vi "TLB Native Dynamic Events ver 0.08d beta.vi"() -> ()   [LabVIEW 2018]
uses:
  Labview Training Phase 2/Enum Controls/States for Action Engine.ctl
  Type def/TLB event states.ctl
  Type def/TLB MHL States.ctl
  <vilib>/Studica/Studica Toolkit/Background/I2C Channel.ctl
  <vilib>/myRIO/Common/Instrument Driver Framework/myRIO v1.0/AI/typedefs/AI Channels Enum.ctl
  <vilib>/myRIO/Common/Instrument Driver Framework/myRIO v1.0/AI/typedefs/AI Channels List.ctl
  Type def/Type def.ctl
  <vilib>/Studica/Studica Blackhawk/Blackhawk.lvlib
  <vilib>/Studica/Studica Toolkit/Background/Mxp Selection.ctl
  <vilib>/Studica/Studica Toolkit/Background/DIO Channel.ctl
  <vilib>/NI_Real-Time Target Support.lvlib
  <vilib>/ptbypt/NI_PtbyPt.lvlib
  <vilib>/addons/control/pid/NI_PID_pid.lvlib
  Underlying VI's/Webcam FGV Low level ver/State control.ctl
  <vilib>/userdefined/High Color/IMAQdx.ctl
  <vilib>/Studica/Studica Toolkit/NavX/NavX.lvlib
  <vilib>/addons/control/pid/pid.llb/PID (DBL).vi
  <vilib>/Studica/Studica Toolkit/NavX/TypeDefs/Flags/Z900_navX_Flags_CalibrationStatusTypeDef.ctl
  <vilib>/Studica/Studica Toolkit/NavX/TypeDefs/Flags/Z900_navX_Flags_OpStatusTypeDef.ctl
panel:
  out "Sensor loop error":errorcluster
  out "Status":T3 {"OP Status" items=["INITIALIZING", "SELFTEST_IN_PROGRESS", "ERROR", "IMU_AUTOCAL_IN_PROGRESS", "NORMAL"]; "Calibration Status" items=["IMU_CAL_STATE_MASK"=3, "IMU_CAL_STATE_INPROGRESS"=0, "IMU_CAL_STATE_ACCUMULATE"=1, "IMU_CAL_STATE_COMPLETE"=2]}
  out "NavX error":errorcluster
  out "Arduino error":errorcluster
  in  "Data to Write":u8[](array[numeric])
  out "Displacement":T4
  out "Yaw":dbl
  out "Speed and distance cluster":T5
  out "Output":dbl
  in  "SENSOR":bool
  out "Decision":i8
  out "Manual Zero Yaw":bool
  in  "error in (no error)":errorcluster
  in  "RED LED State":enum16{"OFF", "ON", "BLINK"}(ring)
  in  "GREEN LED State":enum16{"OFF", "ON", "BLINK"}(ring)
  in  "Red LED":bool
  in  "Green LED":bool
  out "Input state":i8
  out "Waveform Chart 2":dbl(graph)
  out "Waveform Chart":dbl(graph)
  in  "STOP":bool
  out "DIO 0":bool
  out "DIO 1":bool
  out "Limit Switch Array":bool[](array[boolean])
  out "error out":errorcluster
  out "L/R average":fxp<+,64,64>
  out "Right Ultrasonic":fxp<+,64,16>
  out "Left Ultrasonic":fxp<+,64,16>
  out "Right IR Sensor":dbl
  out "Left IR Sensor":dbl
  out "Object detection count":T6
  out "Camera error":errorcluster
  in  "Servo Angle":u8(slide) scale=0.0..180.0
  in  "On/Off":bool
  out "Blackhawk error":errorcluster
  out "element":T7
  out "Action Queue Items":i32
  out "State Logic Queue Items":i32
  out "Action Queues items":string[](array[string])=["Hardware reset", "Software reset", ""]
  out "State logic":T8=enum."Task 2"
  out "Action State":string
  # "TLB FRAMEWORK STATUS"
  # "Camera Status Loop"
  # "Test Programme written by Calvin Loke    Dated: 28 Aug 2019\nTest Programme revised by Dr Alex See   Dated 30 Aug 2019\n\nProgramme version:   TLB Native Dynamic Events ver 0.04b.vi"
  # "Problems now:\nYaw does not work when code is in last state mode\nSlow acceleration due to loop rate?"
  # "Motor Control Loop"
  # "NAVX Control Loop"
  # "Blackhawk status"
  # "Sensor data"
  # "System Health Status Update"
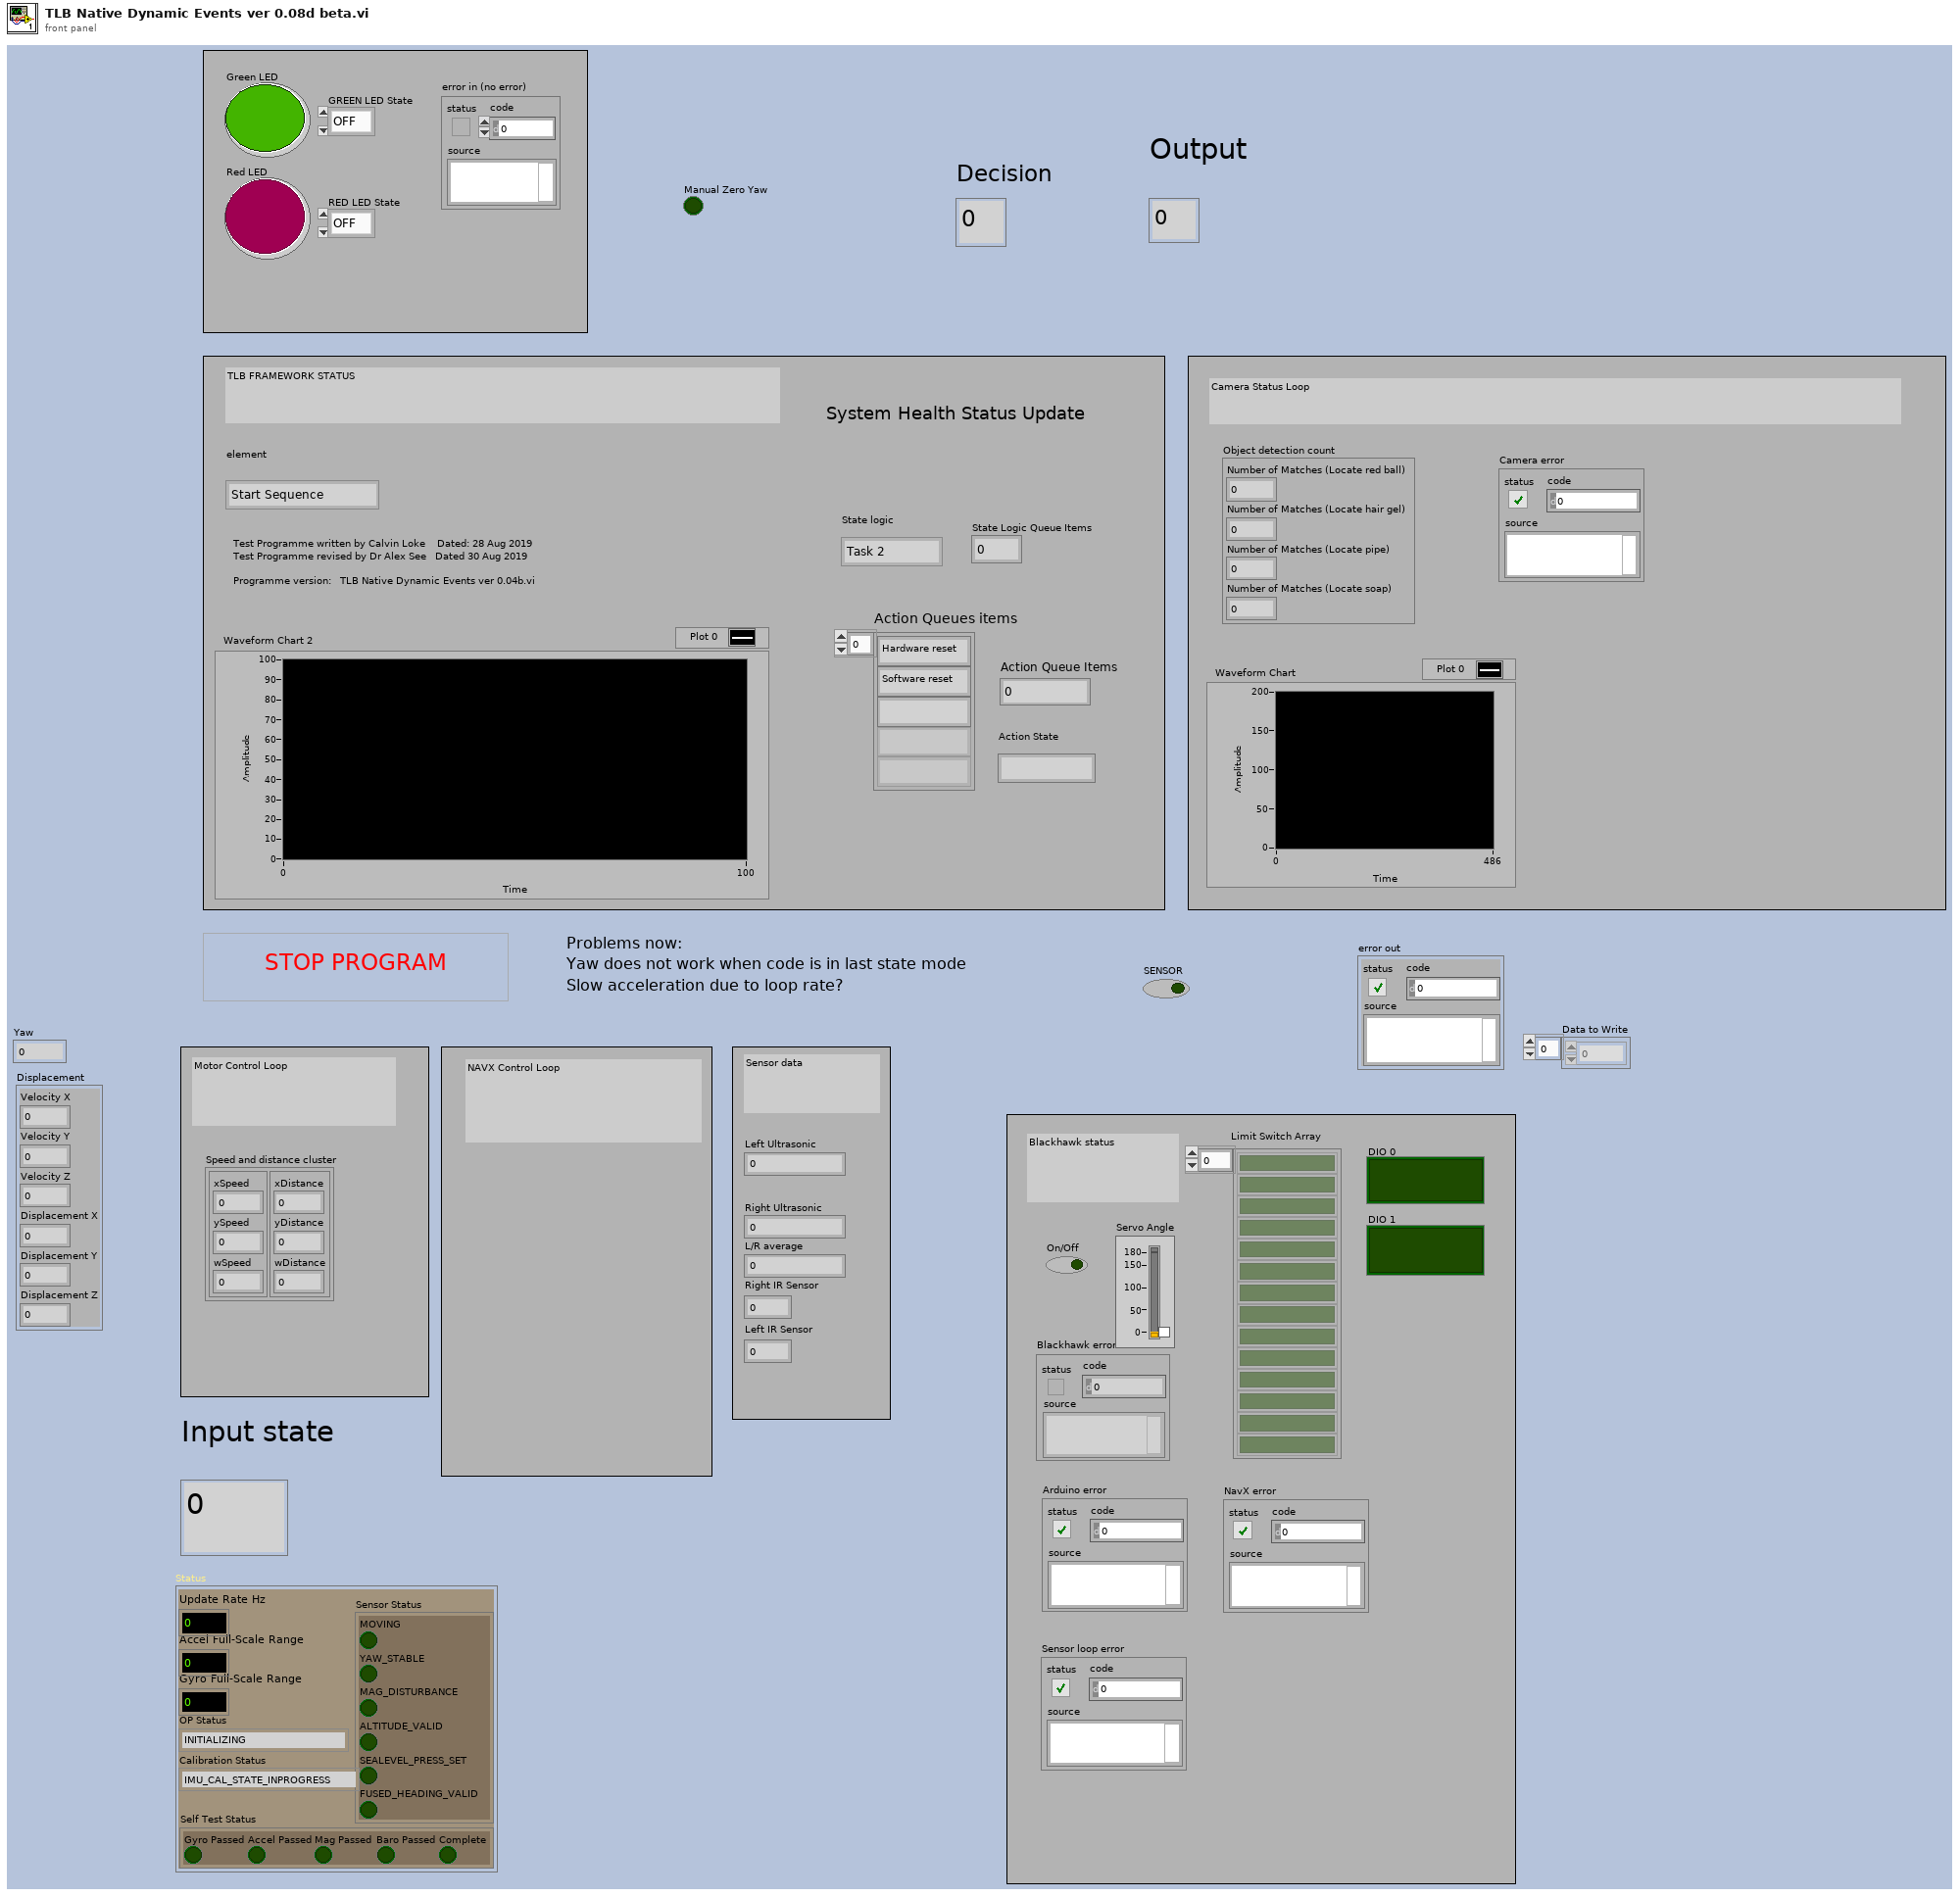
[diagram p1: front panel]
types:
  T1 = typedef "NavX.lvlib/Z900_navX_Flags_OpStatusTypeDef.ctl" = u8
  T2 = typedef "NavX.lvlib/Z900_navX_Flags_CalibrationStatusTypeDef.ctl" = u8
  T3 = cluster{"Update Rate Hz":u8, "Accel Full-Scale Range":u8, "Gyro Full-Scale Range":u16, "OP Status":T1, "Calibration Status":T2, "Sensor Status":cluster{"MOVING":bool, "YAW_STABLE":bool, "MAG_DISTURBANCE":bool, "ALTITUDE_VALID":bool, "SEALEVEL_PRESS_SET":bool, "FUSED_HEADING_VALID":bool}, "Self Test Status":cluster{"Gyro Passed":bool, "Accel Passed":bool, "Mag Passed":bool, "Baro Passed":bool, "Complete":bool}}
  T4 = cluster{"Velocity X":dbl, "Velocity Y":dbl, "Velocity Z":dbl, "Displacement X":dbl, "Displacement Y":dbl, "Displacement Z":dbl}
  T5 = cluster{cluster{"xSpeed":dbl, "ySpeed":dbl, "wSpeed":dbl}, cluster{"xDistance":dbl, "yDistance":dbl, "wDistance":dbl}}
  T6 = cluster{"Number of Matches (Locate red ball)":i32, "Number of Matches (Locate hair gel)":i32, "Number of Matches (Locate pipe)":i32, "Number of Matches (Locate soap)":i32}
  T7 = typedef "TLB event states.ctl" = enum16{"Start Sequence", "Exit", "Start Task 1", "Start Task 2", "Start Task 3", "Start Task 4", "Camera vision", "Wall follow mode", "Idle", "Start Drive Straight"}
  T8 = typedef "TLB MHL States.ctl" = enum16{"None", "Startup", "Idle", "Processing", "Shutdown", "Reset", "Task 1", "Task 2", "Task 3", "Task 4", "Task 4a", "Task 4b", "Task 4c", "Task 4d", "Task 4e", "Task 4f", "Task 4g", "Task 4h", "Acquire image", "Wall follow mode", "Autodrive", "Autodrive a"}
  T9 = typedef "States for Action Engine.ctl" = enum16{"Initialize", "Write", "Read"}
  T10 = typedef "I2C Channel.ctl" = enum16{"Not Connected", "A", "B"}
  T11 = typedef "DIO Channel.ctl" = enum16{"Not Connected", "A/DIO1", "A/DIO2", "A/DIO3", "A/DIO4", "A/DIO5", "A/DIO6", "A/DIO7", "A/DIO13", "B/DIO1", "B/DIO2", "B/DIO3", "B/DIO4", "B/DIO5", "B/DIO6", "B/DIO7", "B/DIO13", "C/DIO0", "C/DIO1", "C/DIO2", "C/DIO3", "C/DIO4", "C/DIO5", "C/DIO6", "C/DIO7"}
  T12 = typedef "Type def.ctl" = cluster{"Front Ultrasonic Obstruct":bool, "Left Ultrasonic Obstruct":bool, "Right Ultrasonic Obstruct ":bool}
  T13 = enum16{"LAST STATE", "STOP", "FORWARD", "BACKWARD", "LEFT", "RIGHT", "RCW", "ACW", "INIT", "RESET ENCODERS"}
  T14 = cluster{"proportional gain (Kc)":dbl, "integral time (Ti, min)":dbl, "derivative time (Td, min)":dbl}
  T15 = typedef "State control.ctl" = enum16{"Initialise", "Start camera", "Continuous Acquisition ", "Stop camera", "Dispose all"}
  T16 = typedef "IMAQdx.ctl" = refnum<k21>
  T17 = typedef "Mxp Selection.ctl" = enum16{"MXP A", "MXP B"}
  T18 = enum16{"DISTANCE READ", "STOP", "FORWARD", "BACKWARD", "LEFT", "RIGHT", "RCW", "ACW", "INIT", "RESET ENCODERS"}
  T19 = typedef "AI Channels List.ctl" = T20[]
  T20 = typedef "AI Channels Enum.ctl" = enum16{"Not Connected", "AudioIn/Left", "AudioIn/Right", "C/AI0", "C/AI1", "A/AI0", "A/AI1", "A/AI2", "A/AI3", "A/AI4", "A/AI5", "A/AI6", "A/AI7", "B/AI0", "B/AI1", "B/AI2", "B/AI3", "B/AI4", "B/AI5", "B/AI6", "B/AI7", "AI/AI0", "AI/AI1", "AI/AI2", "AI/AI3", "A/AI0 (DIFF)", "A/AI1 (DIFF)", "A/AI2 (DIFF)", "A/AI3 (DIFF)", "B/AI0 (DIFF)", "B/AI1 (DIFF)", "B/AI2 (DIFF)", "B/AI3 (DIFF)"}
  T21 = cluster{"I2C Channel":T10, "FPGA VI Reference Out":refnum<k20>}
  T22 = cluster{"DIO Channel":T11, "FPGA VI Reference Out":refnum<k20>}
  T23 = typedef "Analog Scaling Constants List.ctl" = T24[]
  T24 = typedef "Analog Scaling Constants.ctl" = cluster{"LSB Weight (Volts)":dbl, "Offset (Volts)":dbl, "Signed?":bool}
  T25 = cluster{"Scale Constants Array":T23, "FPGA Reference Out":refnum<k20>, "AI Channel":T19}
  T26 = typedef "NI_Real-Time Target Support.lvlib/RT CPU Load.ctl" = cluster{"Total (%)":dbl, "Time Critical (%)":dbl, "Timed Structures (%)":dbl, "High (%)":dbl, "Above Normal (%)":dbl, "Normal (%)":dbl, "Background (%)":dbl, "Idle (%)":dbl, "ISR (%)":dbl}
  T27 = cluster{"CPU loads[0]":T26, "CPU loads[1]":T26, "CPU loads[2]":T26, "CPU loads[3]":T26, "CPU loads[4]":T26, "CPU loads[5]":T26, "CPU loads[6]":T26, "CPU loads[7]":T26, "CPU loads[8]":T26}
  T28 = cluster{"I2C Ref Out":cluster{"I2C Channel":T10, "FPGA VI Reference Out":refnum<k20>}, "Connected":bool, "Slave Address (7-bit)":u8, "Registry":u8[]}
  T29 = typedef "IMAQ Image.ctl" = refnum<image>
  T30 = cluster{"Yaw":dbl, "Roll":dbl, "Pitch":dbl, "Heading":dbl, "Fused Heading":dbl}
  T31 = cluster{"xDistance":dbl, "yDistance":dbl, "wDistance":dbl}
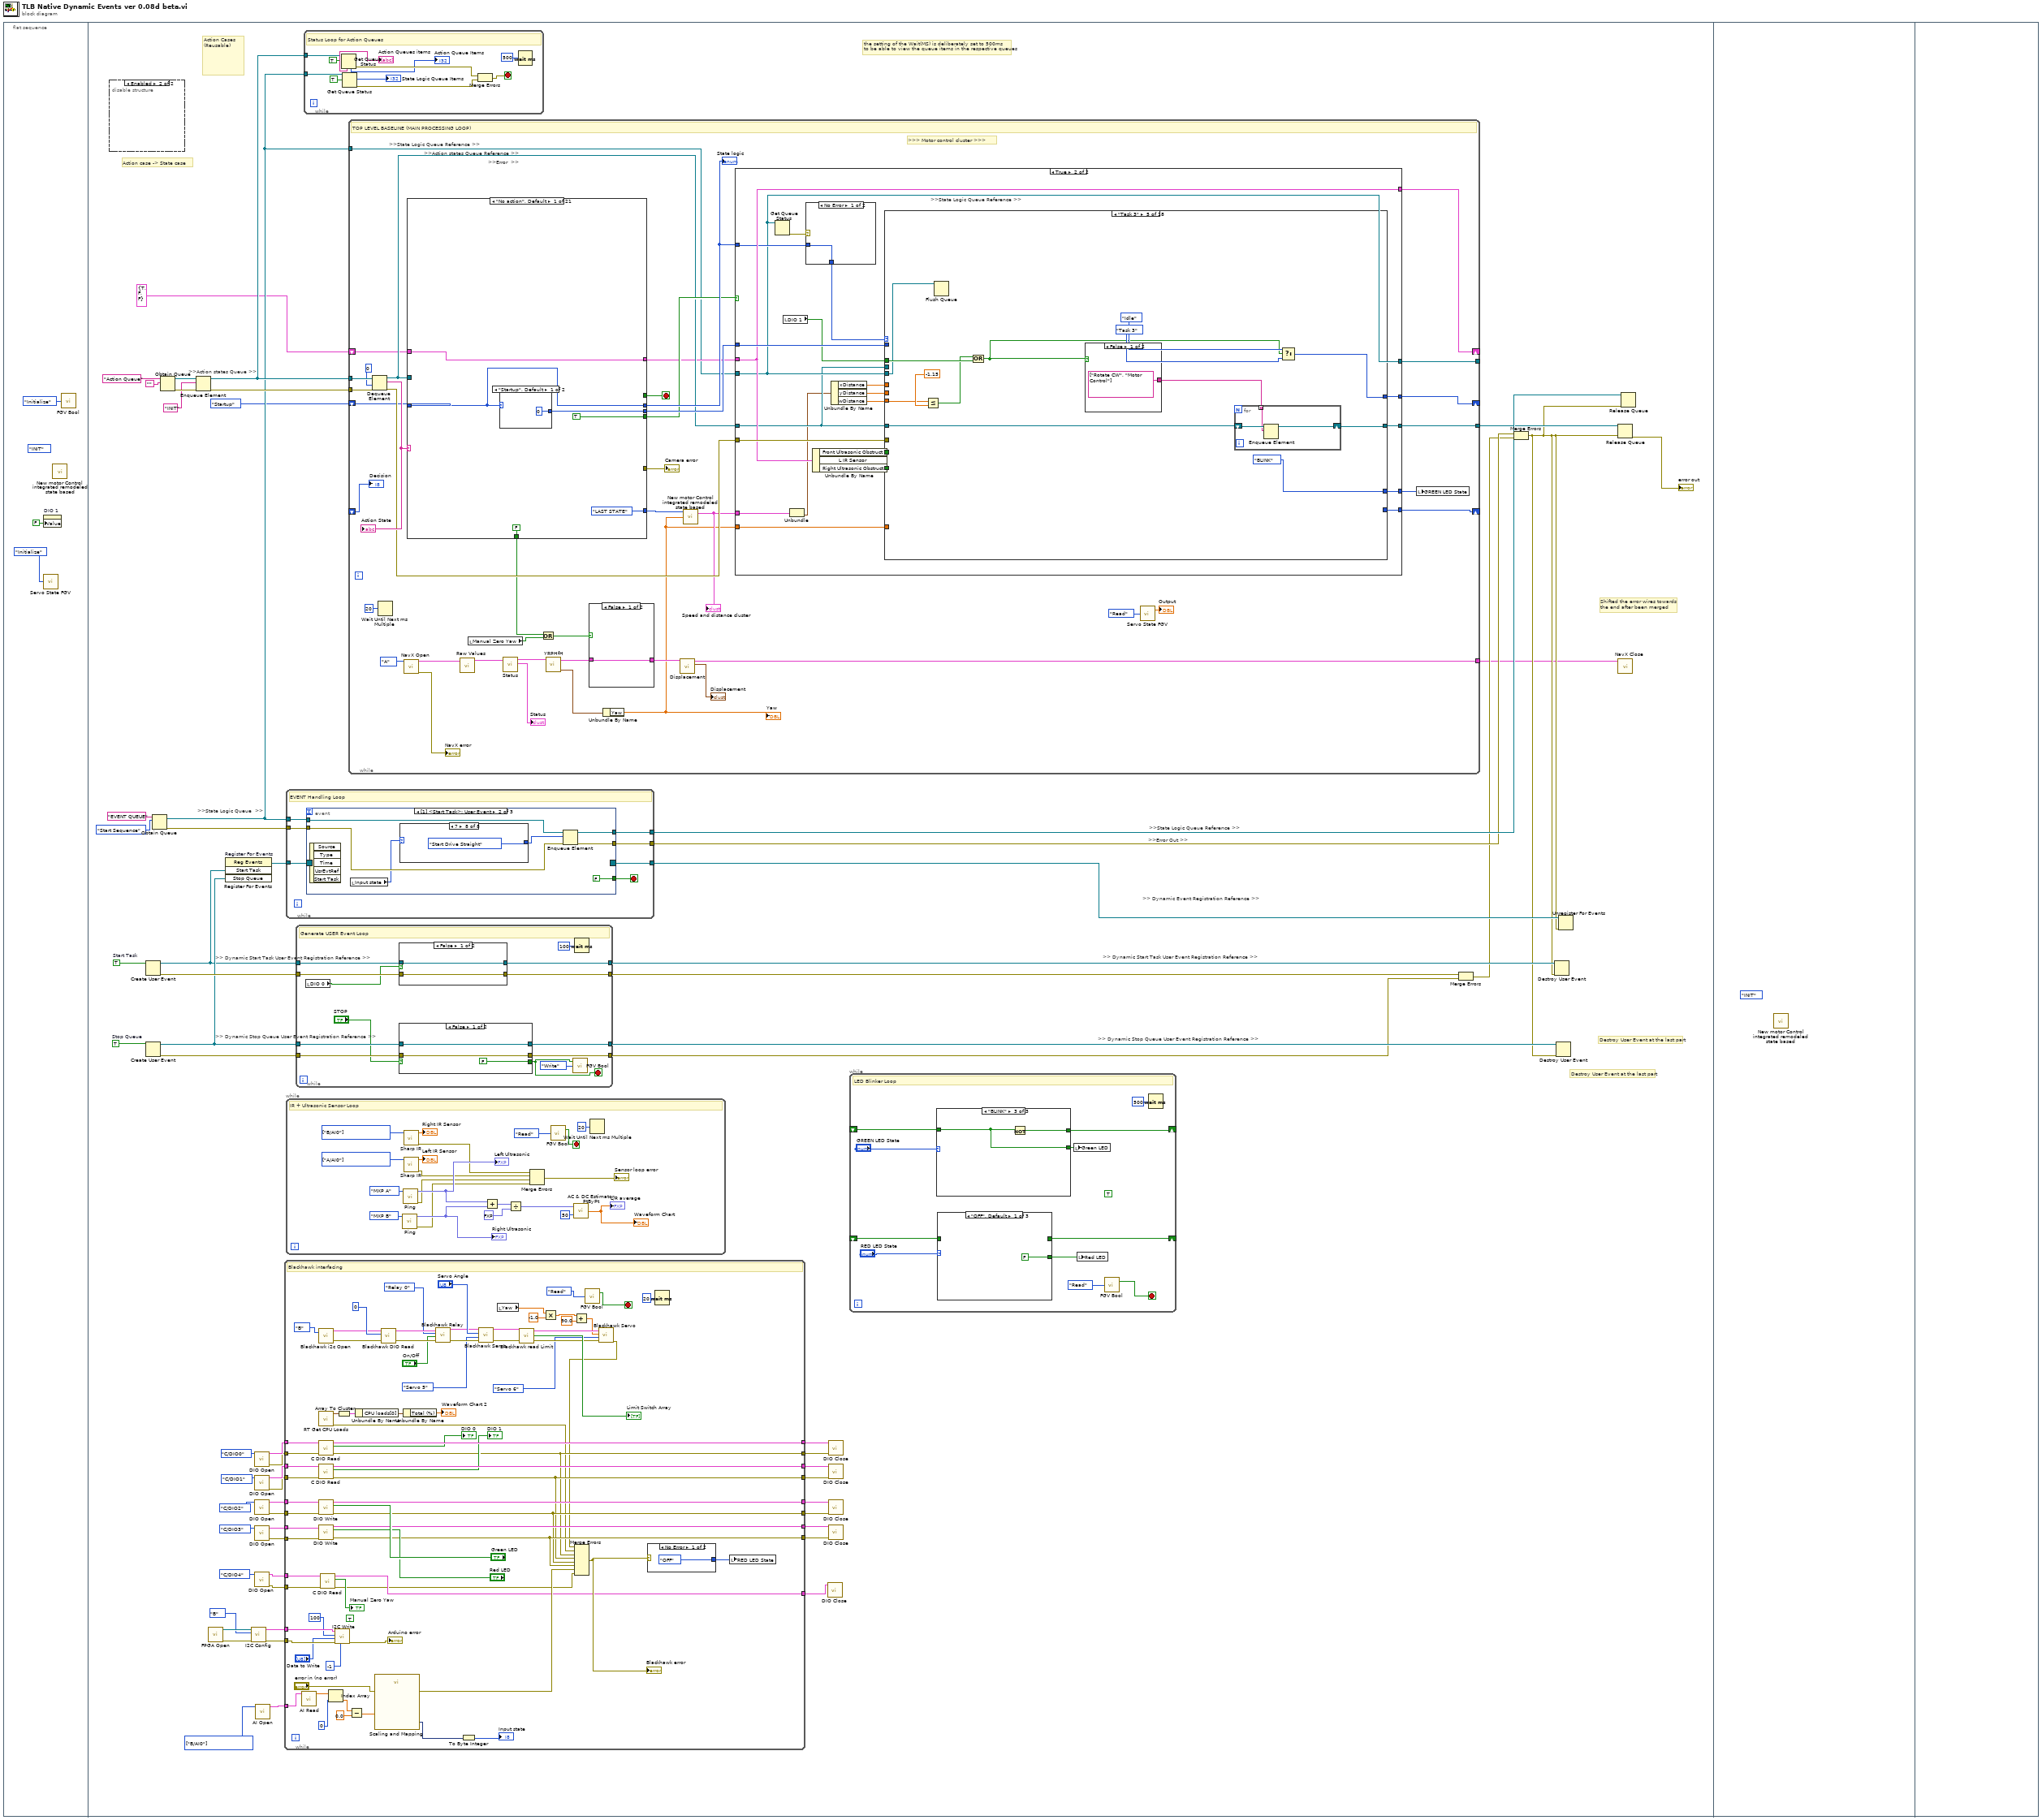
[diagram p0: block diagram]
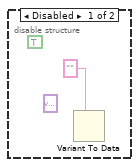
[diagram p2: hidden frame]
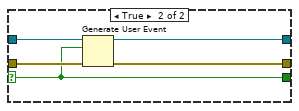
[diagram p3: hidden frame]
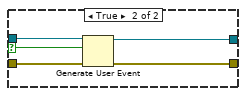
[diagram p4: hidden frame]
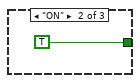
[diagram p5: hidden frame]
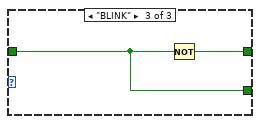
[diagram p6: hidden frame]
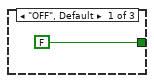
[diagram p7: hidden frame]
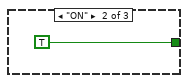
[diagram p8: hidden frame]
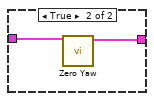
[diagram p9: hidden frame]
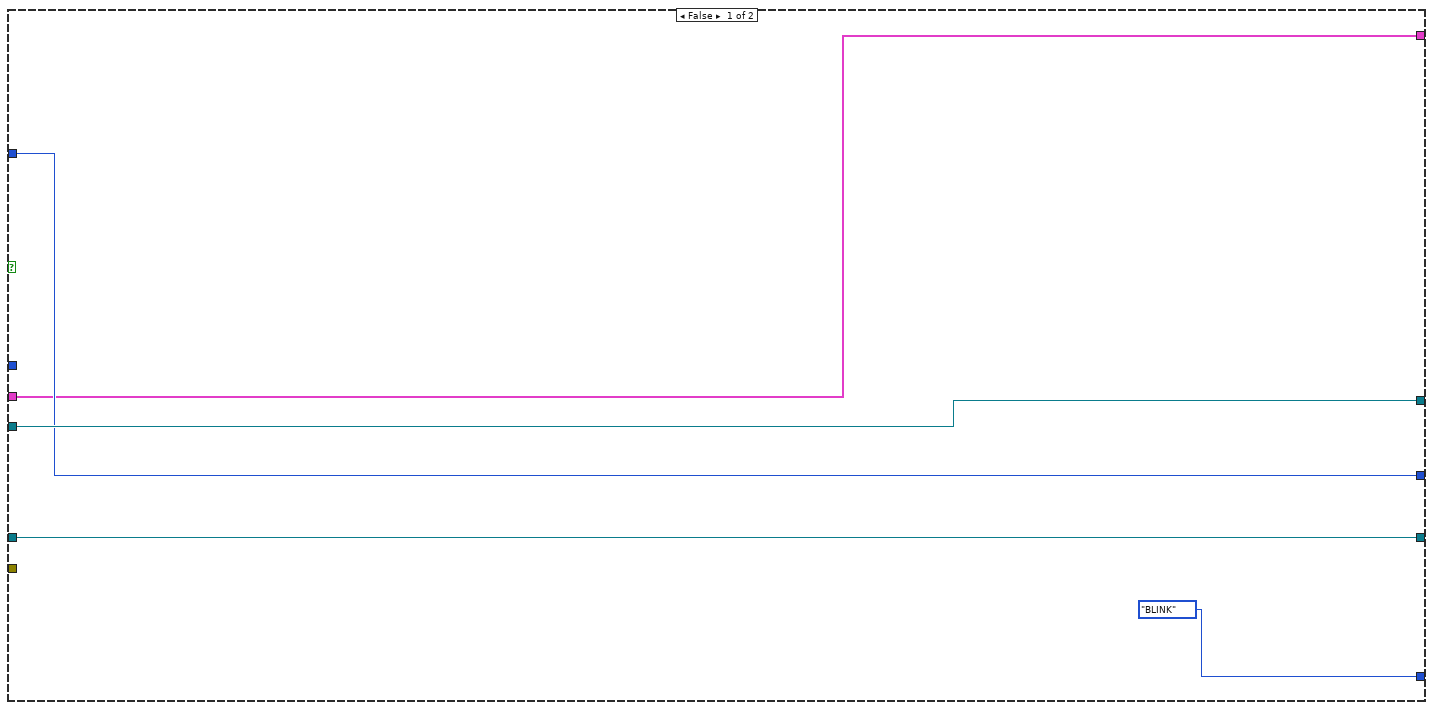
[diagram p10: hidden frame]
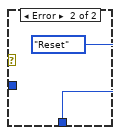
[diagram p11: hidden frame]
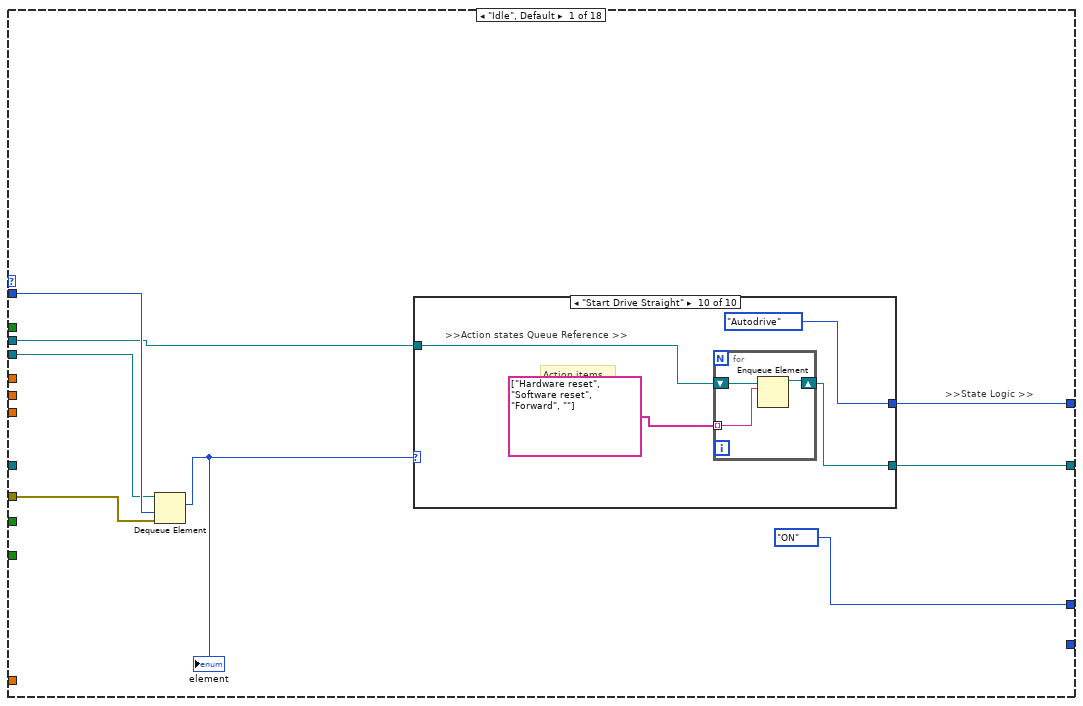
[diagram p12: hidden frame]
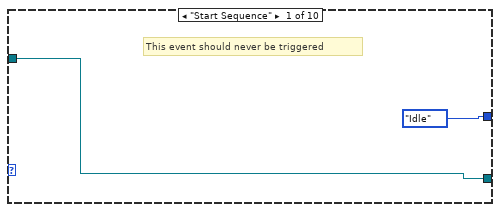
[diagram p13: hidden frame]
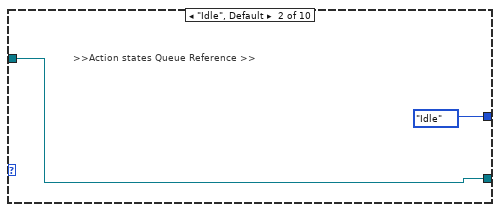
[diagram p14: hidden frame]
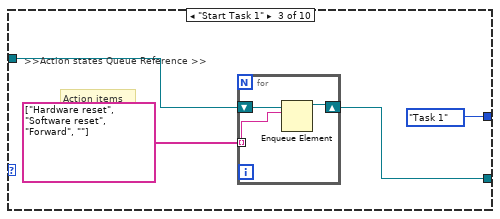
[diagram p15: hidden frame]
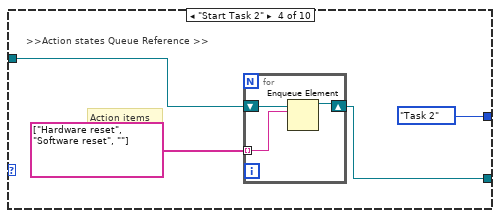
[diagram p16: hidden frame]
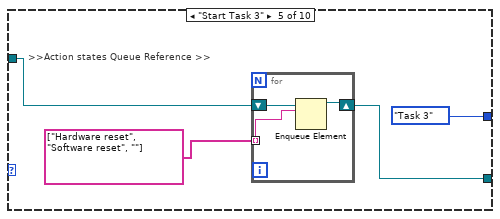
[diagram p17: hidden frame]
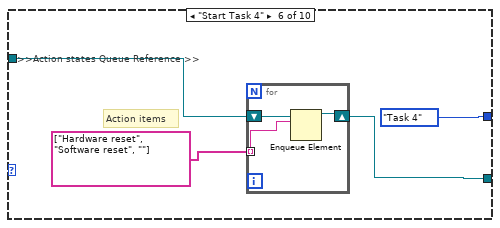
[diagram p18: hidden frame]
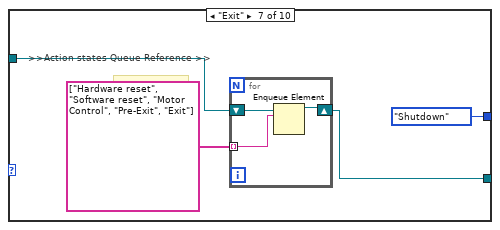
[diagram p19: hidden frame]
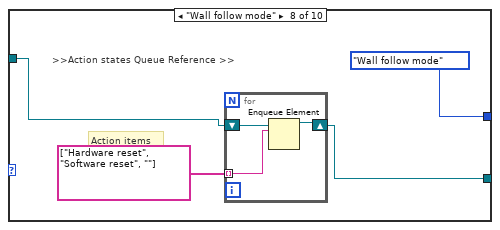
[diagram p20: hidden frame]
diagram:
  n1 = flat-sequence {
    frame #0 {
      (unwired) T18."INIT" ("States")
      n2 = call "Servo State FGV.vi"("Init/Read/Write State"=States_for_Action_Engine."Initialize") -> ()  [unwired: 2 in, 2 out]
      n3 = property on="DIO 1" class="Bool (strict)"("Value"=FALSE ("DIO 1")) -> ()  [unwired: 2 in, 2 out]
      n4 = call "New motor Control integrated remodeled state based.vi"() -> ()  [unwired: 3 in, 2 out]
      n5 = call "FGV Bool.vi"("Init/Read/Write State"=States_for_Action_Engine."Initialize") -> ()  [unwired: 2 in, 2 out]
    }
    frame #1 {
      w19 = T19 [enum."B/AI0"] items=["Not Connected", "AudioIn/Left", "AudioIn/Right", "C/AI0", "C/AI1", "A/AI0", "A/AI1", "A/AI2", "A/AI3", "A/AI4", "A/AI5", "A/AI6", "A/AI7", "B/AI0", "B/AI1", "B/AI2", "B/AI3", "B/AI4", "B/AI5", "B/AI6", "B/AI7", "AI/AI0", "AI/AI1", "AI/AI2", "AI/AI3", "A/AI0 (DIFF)", "A/AI1 (DIFF)", "A/AI2 (DIFF)", "A/AI3 (DIFF)", "B/AI0 (DIFF)", "B/AI1 (DIFF)", "B/AI2 (DIFF)", "B/AI3 (DIFF)"] ("AI Channel")
      w66 = TRUE  # Stop Queue
      w65 = TRUE  # Start Task
      # "Action case -> State case"
      # "the setting of the Wait(MS) is deliberately set to 500ms\nto be able to view the queue items in the respective queues"
      # "Action Cases\n(Reusable)"
      # ">>Error Out >>"
      # ">> Dynamic Stop Queue User Event Registration Reference >>"
      # ">> Dynamic Start Task User Event Registration Reference >>"
      # ">> Dynamic Stop Queue User Event Registration Reference >>"
      # ">> Dynamic Start Task User Event Registration Reference >>"
      # ">> Dynamic Event Registration Reference >>"
      # ">>Action states Queue >>"
      # ">>State Logic Queue  >>"
      # ">>State Logic Queue Reference >>"
      # "Destroy User Event at the last part"
      # "Destroy User Event at the last part"
      # "Shifted the error wires towards\nthe end after been merged"
      n6 = disable-structure shown="Enabled" {
        frame Disabled {
          (unwired) variant
          (unwired) TRUE
          n7 = Variant To Data(type="") -> ()  [unwired: 2 in, 2 out]
        }
        frame Enabled {
        }
      }
      n8 = Create User Event(user event datatype=w65) -> (user event=w57:refnum<user-event>, error out=w62:errorcluster)  [unwired: 1 in]
      n9 = Create User Event(user event datatype=w66) -> (user event=w58:refnum<user-event>, error out=w61:errorcluster)  [unwired: 1 in]
      n10 = Obtain Queue(name (unnamed)="EVENT QUEUE", element data type=TLB_event_states."Start Sequence" ("Enum")) -> (queue out=w42:refnum<queue>, error out=w48:errorcluster)  [unwired: 3 in, 1 out]
      n11 = Obtain Queue(name (unnamed)="Action Queue", element data type="") -> (queue out=w51:refnum<queue>, error out=w47:errorcluster)  [unwired: 3 in, 1 out]
      n12 = Enqueue Element(queue=w51, element="INIT", error in (no error)=w47) -> (queue out=w43:refnum<queue>, error out=w46:errorcluster)  [unwired: 1 in, 1 out]
      n13 = call <vilib>:"FPGA Open.vi"() -> ("error out"=w8:errorcluster, "FPGA Reference Out"=w9:refnum<k20>)  [unwired: 10 in]
      n14 = register-events "Register For Events"(w57, w58) -> (reference out=w56:refnum<event-registration>)  [unwired: 2 in, 1 out]
      n15 = call <vilib>:"I2C Config.vi"("error in (no error)"=w8, "I2C Channel"=I2C_Channel."B", "FPGA Reference"=w9) -> ("error out"=w7:errorcluster, "I2C Ref Out"=w4:T21)  [unwired: 7 in]
      n16 = call <vilib>:"DIO Open.vi"("DIO Channel"=DIO_Channel."C/DIO4") -> ("error out"=w5:errorcluster, "DIO Info Out"=w13:T22)  [unwired: 9 in]
      n17 = call <vilib>:"DIO Open.vi"("DIO Channel"=DIO_Channel."C/DIO0") -> ("error out"=w29:errorcluster, "DIO Info Out"=w35:T22)  [unwired: 9 in]
      n18 = call <vilib>:"DIO Open.vi"("DIO Channel"=DIO_Channel."C/DIO1") -> ("error out"=w27:errorcluster, "DIO Info Out"=w31:T22)  [unwired: 9 in]
      n19 = call <vilib>:"DIO Open.vi"("DIO Channel"=DIO_Channel."C/DIO2") -> ("error out"=w17:errorcluster, "DIO Info Out"=w23:T22)  [unwired: 9 in]
      n20 = call <vilib>:"DIO Open.vi"("DIO Channel"=DIO_Channel."C/DIO3") -> ("error out"=w15:errorcluster, "DIO Info Out"=w22:T22)  [unwired: 9 in]
      n21 = call <vilib>:"AI Open.vi"("AI Channel"=w19) -> ("Analog Info"=w18:T25)  [unwired: 9 in, 1 out]
      n22 = while {
        tunnel: w35 -> [w758]
        tunnel: [w757] -> w34
        tunnel: w31 -> [w756]
        tunnel: [w755] -> w30
        tunnel: w29 -> [w754]
        tunnel: [w723] -> w28
        tunnel: w27 -> [w753]
        tunnel: [w724] -> w26
        tunnel: w23 -> [w747]
        tunnel: w22 -> [w746]
        tunnel: [w743] -> w21
        tunnel: [w742] -> w20
        tunnel: w18 -> [w741]
        tunnel: w17 -> [w734]
        tunnel: [w725] -> w16
        tunnel: w15 -> [w733]
        tunnel: [w726] -> w14
        tunnel: w13 -> [w714]
        tunnel: [w713] -> w11
        tunnel: w7 -> [w704]
        tunnel: w5 -> [w706]
        tunnel: w4 -> [w702]
        stop <- w771 stop-if-true
        (unwired) TRUE ("Keep Bus Busy")
        # "Blackhawk interfacing"
        n23 = call <vilib>:"AI Read.vi"("Analog Info"=w741) -> ("Array"=w737:dbl[])  [unwired: 9 in, 1 out]
        n24 = call <vilib>:"Blackhawk i2c Open.vi"("I2C Channel"=I2C_Channel."B") -> ("I2C Ref Out"=w749:T21, "error out"=w748:errorcluster)  [unwired: 2 in]
        n25 = call <vilib>:"RT Get CPU Loads.vi"() -> ("error out"=w722:errorcluster, "CPU loads"=w728:T26[])  [unwired: 10 in]
        n26 = call <vilib>:"C DIO Read.vi"("error in (no error)"=w754, "DIO Info In in"=w758) -> ("error out"=w723:errorcluster, "IN"=→"DIO 0":bool, "DIO Info In out"=w757:T22)  [unwired: 7 in]
        n27 = call <vilib>:"C DIO Read.vi"("error in (no error)"=w753, "DIO Info In in"=w756) -> ("error out"=w724:errorcluster, "IN"=→"DIO 1":bool, "DIO Info In out"=w755:T22)  [unwired: 7 in]
        n28 = call <vilib>:"DIO Write.vi"("error in (no error)"=w734, "Input"="Green LED", "DIO Info In"=w747) -> ("error out"=w725:errorcluster, "DIO Info Out"=w743:T22)  [unwired: 7 in]
        n29 = call <vilib>:"DIO Write.vi"("error in (no error)"=w733, "Input"="Red LED", "DIO Info In"=w746) -> ("error out"=w726:errorcluster, "DIO Info Out"=w742:T22)  [unwired: 7 in]
        n30 = call <vilib>:"C DIO Read.vi"("error in (no error)"=w706, "DIO Info In in"=w714) -> ("error out"=w705:errorcluster, "IN"=→"Manual Zero Yaw":bool, "DIO Info In out"=w713:T22)  [unwired: 7 in]
        n31 = Index Array(array=w737, index=0) -> (element=w739:dbl)
        n32 = call <vilib>:"I2C Write.vi"("Timeout ms (1000)"=-1, "error in (no error)"=w704, "Data to Write"="Data to Write", "Slave Address (7-bit)"=u8 100, "I2C Ref In"=w702) -> ("error out"=→"Arduino error":errorcluster)  [unwired: 5 in, 1 out]
        n33 = Array To Cluster(array=w728) -> (cluster=w729:T27)
        n34 = Subtract(x=w739, y=0.0) -> (x-y=w740:dbl)
        n35 = Unbundle By Name(w729) -> ("CPU loads[0]"=w730:T26)
        n36 = call "Scaling and Mapping"("error in (no error)"="error in (no error)", "Signals"=w740) -> ("error out"=w727:errorcluster, "Scaled Signals"=w735:dynamicdata)  [unwired: 8 in]
        n37 = call <vilib>:"Blackhawk DIO Read.vi"("I2C Ref In"=w749, "PIN"=u8 0, "error in (no error)"=w748) -> ("I2C Ref Out"=w769:T21, "error out"=w770:errorcluster)  [unwired: 3 in, 1 out]
        n38 = Unbundle By Name(w730) -> ("Total (%)"=→"Waveform Chart 2":dbl)
        n39 = call <vilib>:"Blackhawk Relay.vi"("error in (no error)"=w770, "On/Off"="On/Off", "Relay"=enum8{"Relay 0", "Relay 1", "Relay 2"}."Relay 0", "I2C Ref In"=w769) -> ("error out"=w766:errorcluster, "I2C Ref Out"=w763:T21)  [unwired: 6 in]
        n40 = To Byte Integer(number=w735) -> (8bit integer=→"Input state":i8)
        n41 = call <vilib>:"Blackhawk Servo.vi"("error in (no error)"=w766, "Servo Select"=enum16{"Servo 5", "Servo 6"}."Servo 5", "Servo Angle"="Servo Angle", "I2C Ref In"=w763) -> ("error out"=w761:errorcluster, "I2C Ref Out"=w760:T21)  [unwired: 6 in]
        n42 = local read "Yaw"() -> (w707:dbl)
        n43 = call <vilib>:"Blackhawk read Limit.vi"("error in (no error)"=w761, "I2C Ref In"=w760) -> ("error out"=w718:errorcluster, "Limit Switch Array"=→"Limit Switch Array":bool[], "I2C Ref Out"=w716:T21)  [unwired: 1 in]
        n44 = Multiply(x=w707, y=-1.0) -> (x*y=w709:dbl)
        n45 = Add(x=w709, y=90.0) -> (x+y=w710:dbl)
        n46 = call "FGV Bool.vi"("Init/Read/Write State"=States_for_Action_Engine."Read") -> ("Output node"=w771:bool)  [unwired: 2 in, 1 out]
        n47 = call <vilib>:"Blackhawk Servo.vi"("error in (no error)"=w718, "Servo Select"=enum16{"Servo 5", "Servo 6"}."Servo 6", "Servo Angle"=w710, "I2C Ref In"=w716) -> ("error out"=w717:errorcluster)  [unwired: 6 in, 1 out]
        n48 = Merge Errors(w717, w722, w723, w724, w725, w726, w727, w705) -> (w721:errorcluster)
        "Blackhawk error" <- w721
        n49 = case shown="No Error" w721 {
          tunnel: [enum16{"OFF", "ON", "BLINK"}."OFF" ("RED LED State") enum16{"OFF", "ON", "BLINK"}."BLINK" ("RED LED State")] -> w732
          frame No Error {
          }
          frame Error {
          }
        }
        n50 = Wait (ms)(milliseconds to wait=u32 20) -> ()  [unwired: 1 out]
        n51 = local write "RED LED State"(w732) -> ()
      }
      n52 = while {
        tunnel: w56 -> [w671]
        tunnel: [w670] -> w55
        tunnel: w42 -> [w668]
        tunnel: [w667] -> w54
        tunnel: w48 -> [w666]
        tunnel: [w665] -> w45
        stop <- w669 stop-if-true
        # "EVENT Handling Loop"
        n53 = event shown="[1] <Start Task>: User Event" {
          selector: w671 -> [_ _ _]
          dyn-events: [_ _ _] -> w670
          timeout: _ -> [_ _ _]
          tunnel: [FALSE FALSE w698] -> w669
          tunnel: w668 -> [w676 w683 w696]
          tunnel: [w675 w682 w697] -> w667
          tunnel: w666 -> [w673 w681 w694]
          tunnel: [w672 w680 w693] -> w665
          event Timeout {
            n54 = event-data() -> ()  [unwired: 1 in, 3 out]
            n55 = Enqueue Element(queue=w676, element=TLB_event_states."Idle" ("Enum"), error in (no error)=w673) -> (queue out=w675:refnum<queue>, error out=w672:errorcluster)  [unwired: 1 in, 1 out]
          }
          event User Event {
            n56 = event-data() -> ()  [unwired: 1 in, 5 out]
            n57 = local read "Input state"() -> (w679:i8)
            n58 = case shown="7" w679 {
              tunnel: [TLB_event_states."Idle" ("Enum") TLB_event_states."Start Task 1" ("Enum") TLB_event_states."Start Task 2" ("Enum") TLB_event_states."Start Task 3" ("Enum") TLB_event_states."Start Task 4" ("Enum") TLB_event_states."Wall follow mode" ("Enum") TLB_event_states."Camera vision" ("Enum") TLB_event_states."Start Drive Straight" ("Enum")] -> w678
              frame 0 {
              }
              frame 1 {
              }
              frame 2 {
              }
              frame 3, Default {
              }
              frame 4 {
              }
              frame 5 {
              }
              frame 6 {
              }
              frame 7 {
              }
            }
            n59 = Enqueue Element(queue=w683, element=w678, error in (no error)=w681) -> (queue out=w682:refnum<queue>, error out=w680:errorcluster)  [unwired: 1 in, 1 out]
          }
          event User Event {
            n60 = event-data() -> ("Stop Queue"=w698:bool)  [unwired: 1 in, 4 out]
            n61 = Enqueue Element At Opposite End(queue=w696, element=TLB_event_states."Exit" ("Enum"), error in (no error)=w694) -> (queue out=w697:refnum<queue>, error out=w693:errorcluster)  [unwired: 1 in, 1 out]
          }
        }
      }
      n62 = while {
        stop <- w658 stop-if-true
        w663 = T19 [enum."A/AI0"] items=["Not Connected", "AudioIn/Left", "AudioIn/Right", "C/AI0", "C/AI1", "A/AI0", "A/AI1", "A/AI2", "A/AI3", "A/AI4", "A/AI5", "A/AI6", "A/AI7", "B/AI0", "B/AI1", "B/AI2", "B/AI3", "B/AI4", "B/AI5", "B/AI6", "B/AI7", "AI/AI0", "AI/AI1", "AI/AI2", "AI/AI3", "A/AI0 (DIFF)", "A/AI1 (DIFF)", "A/AI2 (DIFF)", "A/AI3 (DIFF)", "B/AI0 (DIFF)", "B/AI1 (DIFF)", "B/AI2 (DIFF)", "B/AI3 (DIFF)"] ("AI Channel")
        w664 = T19 [enum."B/AI0"] items=["Not Connected", "AudioIn/Left", "AudioIn/Right", "C/AI0", "C/AI1", "A/AI0", "A/AI1", "A/AI2", "A/AI3", "A/AI4", "A/AI5", "A/AI6", "A/AI7", "B/AI0", "B/AI1", "B/AI2", "B/AI3", "B/AI4", "B/AI5", "B/AI6", "B/AI7", "AI/AI0", "AI/AI1", "AI/AI2", "AI/AI3", "A/AI0 (DIFF)", "A/AI1 (DIFF)", "A/AI2 (DIFF)", "A/AI3 (DIFF)", "B/AI0 (DIFF)", "B/AI1 (DIFF)", "B/AI2 (DIFF)", "B/AI3 (DIFF)"] ("AI Channel")
        # "IR + Ultrasonic Sensor Loop"
        n63 = call <vilib>:"Ping.vi"("Mxp Side"=Mxp_Selection."MXP B") -> ("error out"=w647:errorcluster, "CM"=w652:fxp<+,64,16>)  [unwired: 8 in, 1 out]
        "Right Ultrasonic" <- w652
        n64 = call <vilib>:"Ping.vi"("Mxp Side"=Mxp_Selection."MXP A") -> ("error out"=w648:errorcluster, "CM"=w653:fxp<+,64,16>)  [unwired: 8 in, 1 out]
        "Left Ultrasonic" <- w653
        n65 = call <vilib>:"Sharp IR.vi"("AI Channel"=w664) -> ("error out"=w645:errorcluster, "Sharp IR Distance"=→"Right IR Sensor":dbl)  [unwired: 8 in, 1 out]
        n66 = call <vilib>:"Sharp IR.vi"("AI Channel"=w663) -> ("error out"=w646:errorcluster, "Sharp IR Distance"=→"Left IR Sensor":dbl)  [unwired: 8 in, 1 out]
        n67 = Add(x=w653, y=w652) -> (x+y=w655:fxp<+,64,17>)
        n68 = Divide(x=w655, y=fxp<+,64,17> 2.0) -> (x/y=w651:fxp<+,64,64>)
        n69 = Merge Errors(w645, w646, w648, w647) -> (→"Sensor loop error":errorcluster)
        n70 = call "FGV Bool.vi"("Init/Read/Write State"=States_for_Action_Engine."Read") -> ("Output node"=w658:bool)  [unwired: 2 in, 1 out]
        n71 = call <vilib>:"AC & DC Estimator PtByPt.vi"("signal"=w651, "sample length"=50) -> ("DC estimate (V)"=→"L/R average" →"Waveform Chart":dbl)  [unwired: 1 in, 2 out]
        n72 = Wait Until Next ms Multiple(millisecond multiple=u32 20) -> ()  [unwired: 1 out]
      }
      n73 = while {
        tunnel: w57 -> [w90]
        tunnel: w58 -> [w89]
        tunnel: [w88] -> w64
        tunnel: [w87] -> w63
        tunnel: w62 -> [w86]
        tunnel: [w85] -> w60
        tunnel: w61 -> [w84]
        tunnel: [w83] -> w59
        stop <- w81 stop-if-true
        # "Generate USER Event Loop"
        n74 = local read "DIO 0"() -> (w80:bool)
        n75 = case shown="False" w80 {
          selector: w80 -> [_ w102]
          tunnel: w90 -> [w101 w106]
          tunnel: [w101 w105] -> w87
          tunnel: w86 -> [w100 w104]
          tunnel: [w100 w103] -> w85
          frame False {
          }
          frame True {
            n76 = Generate User Event(user event=w106, event data cluster=w102, error in=w104) -> (user event out=w105:refnum<user-event>, error out=w103:errorcluster)  [unwired: 1 in]
          }
        }
        n77 = case shown="False" "STOP" {
          selector: "STOP" -> [_ w95]
          tunnel: w89 -> [w94 w99]
          tunnel: [w94 w98] -> w88
          tunnel: w84 -> [w93 w97]
          tunnel: [w93 w96] -> w83
          tunnel: [FALSE w95] -> w81
          frame False {
          }
          frame True {
            n78 = Generate User Event(user event=w99, event data cluster=w95, error in=w97) -> (user event out=w98:refnum<user-event>, error out=w96:errorcluster)  [unwired: 1 in]
          }
        }
        n79 = call "FGV Bool.vi"("Init/Read/Write State"=States_for_Action_Engine."Write", "Input Node"=w81) -> ()  [unwired: 1 in, 2 out]
        n80 = Wait (ms)(milliseconds to wait=u32 100) -> ()  [unwired: 1 out]
      }
      n81 = while {
        tunnel: w43 -> [w76]
        tunnel: w42 -> [w73]
        stop <- w70 stop-if-true
        # "Status Loop for Action Queues"
        n82 = Get Queue Status(queue=w76, return elements? (F)=TRUE) -> (error out=w72:errorcluster, # elements in queue=→"Action Queue Items":i32, elements=→"Action Queues items":string[])  [unwired: 1 in, 5 out]
        n83 = Get Queue Status(queue=w73, return elements? (F)=TRUE) -> (# pending remove=→"State Logic Queue Items":i32, error out=w71:errorcluster)  [unwired: 1 in, 6 out]
        n84 = Merge Errors(w72, w71) -> (w70:errorcluster)
        n85 = Wait (ms)(milliseconds to wait=u32 500) -> ()  [unwired: 1 out]
      }
      n86 = while {
        tunnel: w42 -> [w150]
        shift-right: [w161] -> _
        shift-left: TLB_MHL_States."Startup" ("Enum") -> [w155]
        tunnel: w43 -> [w166]
        tunnel: w46 -> [w164]
        tunnel: [w163] -> _
        tunnel: [w162] -> w38
        shift-right: [w152] -> _
        shift-left: T12 {"Front Ultrasonic Obstruct"=TRUE, "Left Ultrasonic Obstruct"=FALSE, "Right Ultrasonic Obstruct "=FALSE} -> [w154]
        shift-right: [w144] -> _
        shift-left: _ -> [w143]
        tunnel: [w133] -> w10
        stop <- w148 stop-if-true
        # ">>> Motor control cluster >>>"
        # ">>Error  >>"
        # ">>Action states Queue Reference >>"
        # ">>State Logic Queue Reference >>"
        # "TOP LEVEL BASELINE (MAIN PROCESSING LOOP)"
        n87 = Dequeue Element(queue=w166, timeout in ms (-1)=0, error in (no error)=w164) -> (queue out=w156:refnum<queue>, element=w165:string, error out=w157:errorcluster)  [unwired: 1 out]
        "Action State" <- w165
        n88 = Wait Until Next ms Multiple(millisecond multiple=u32 20) -> ()  [unwired: 1 out]
        n89 = call <vilib>:"NavX Open.vi"("I2C Channel"=I2C_Channel."A") -> ("error out"=→"NavX error":errorcluster, "NavX Info"=w137:T28)  [unwired: 9 in]
        n90 = case shown="\"No action\", Default" w165 {
          tunnel: [w498 w513 w519 w524 w529 w535 w540 w543 w550 w555 w565 w572 TLB_MHL_States."Shutdown" ("Enum") w582 w593 w596 w607 w618 w626 w638 w642] -> w167
          tunnel: [w501 0 0 0 0 0 0 0 0 0 0 0 0 0 0 0 0 0 0 0 0] -> w160
          tunnel: [TRUE FALSE FALSE FALSE FALSE FALSE FALSE FALSE FALSE FALSE FALSE FALSE FALSE FALSE FALSE FALSE FALSE FALSE FALSE FALSE FALSE] -> w159
          tunnel: w156 -> [_ _ _ _ _ _ _ _ _ _ _ _ _ _ _ _ _ _ _ _ _]
          tunnel: w155 -> [w498 w513 w519 w524 w529 w535 w540 w543 w550 w555 w565 w572 _ w582 w593 w596 w607 w618 w626 w638 w642]
          tunnel: w154 -> [w499 w508 w516 w525 w527 w532 w537 w542 w547 w553 w562 w569 w575 w583 w592 w599 w608 w619 w625 w635 w643]
          tunnel: [w499 w507 w515 w525 w527 w532 w537 w542 w547 w553 w561 w569 w575 w583 w589 w598 w608 w619 w625 w635 w643] -> w153
          tunnel: [_ _ _ _ _ _ _ _ _ _ _ _ _ _ _ _ _ w609 w621 w629 _] -> w151
          tunnel: [_ _ _ _ _ _ _ _ _ _ _ _ TRUE _ _ _ _ _ _ _ _] -> w148
          tunnel: [T13."LAST STATE" ("Move mode") T13."INIT" ("Move mode") T13."FORWARD" ("Move mode") T13."LAST STATE" ("Move mode") T13."BACKWARD" ("Move mode") T13."RIGHT" ("Move mode") T13."LEFT" ("Move mode") T13."RCW" ("Move mode") T13."ACW" ("Move mode") T13."STOP" ("Move mode") _ T13."RESET ENCODERS" ("Move mode") T13."INIT" ("Move mode") T13."INIT" ("Move mode") _ _ _ _ _ _ _] -> w146
          tunnel: [FALSE ("NavX Zero Yaw") _ _ _ _ _ _ _ _ FALSE ("NavX Zero Yaw") FALSE ("NavX Zero Yaw") TRUE ("NavX Zero Yaw") _ _ _ _ _ _ _ _ _] -> w130
          frame "No action", Default {
            n91 = case shown="\"Startup\", Default" w498 {
              tunnel: [0 100] -> w501
              frame "Startup", Default {
              }
              frame "Idle" {
              }
            }
          }
          frame "Init" {
            # ">>State Logic  >>"
            n92 = local write "Servo Angle"(u8 90 ("Servo Angle")) -> ()
            n93 = Bundle By Name(cluster=w508, "Front Ultrasonic Obstruct"=FALSE ("Object detected"), "L IR Sensor"=0.0, "Right Ultrasonic Obstruct"=FALSE ("In move state?")) -> (w507:T12)
          }
          frame "Forward" {
            n94 = Bundle By Name(cluster=w516, "Right Ultrasonic Obstruct"=TRUE ("In move state?")) -> (w515:T12)
          }
          frame " Motor Control" {
          }
          frame "Reverse" {
          }
          frame "Right" {
          }
          frame "Left" {
          }
          frame "Rotate CW" {
          }
          frame "Rotate ACW" {
          }
          frame "Stop" {
          }
          frame "Software reset" {
            w557 = FALSE ("In move state?")
            # "Resets any software variables\nand/or non-critical states"
            n95 = Wait (ms)(milliseconds to wait=u32 20) -> ()  [unwired: 1 out]
            n96 = Bundle By Name(cluster=w562, "Front Ultrasonic Obstruct"=w557, "L IR Sensor"=0.0, "Right Ultrasonic Obstruct"=w557) -> (w561:T12)
          }
          frame "Hardware reset" {
            n97 = Wait (ms)(milliseconds to wait=u32 100) -> ()  [unwired: 1 out]
          }
          frame "Exit" {
          }
          frame "Pre-Exit" {
          }
          frame "Ultrasonic read" {
            # "Object detection"
            n98 = local read "L/R average"() -> (w587:fxp<+,64,64>)
            n99 = Less Or Equal?(x=w587, y=35.0) -> (x <= y?=w586:bool)
            n100 = Or(x=w586, y="SENSOR") -> (x .or. y?=w585:bool)
            n101 = Bundle By Name(cluster=w592, "Front Ultrasonic Obstruct"=w585) -> (w589:T12)
          }
          frame "IR Sensor Read" {
            n102 = local read "Left IR Sensor"() -> (w597:dbl)
            n103 = Bundle By Name(cluster=w599, "L IR Sensor"=w597) -> (w598:T12)
          }
          frame "Calculate" {
            n104 = Unbundle By Name(w608) -> ("L IR Sensor"=w603:dbl)
            n105 = call-poly <vilib>:"PID.vi"("output range"=cluster{"output high":dbl, "output low":dbl} {"output high"=0.3, "output low"=-0.3}, "PID gains"=T14 {"proportional gain (Kc)"=0.01, "integral time (Ti, min)"=0.0, "derivative time (Td, min)"=0.0}, "process variable"=w603, "setpoint"=20.0) -> ("output"=w600:dbl)  [unwired: 6 in, 1 out]
            n106 = Negate(x=w600) -> ()  [unwired: 1 out]
          }
          frame "Cam Init" {
            n107 = call "Low-Level Grab.vi"("States"=State_control."Initialise", "Session In"=T16 "cam1") -> ("error out"=w610:errorcluster, "Session Out"=w611:T16)  [unwired: 7 in, 1 out]
            n108 = call "Low-Level Grab.vi"("error in (no error)"=w610, "States"=State_control."Start camera", "Session In"=w611) -> ("error out"=w609:errorcluster)  [unwired: 6 in, 2 out]
            n109 = local write "Servo Angle"(u8 170 ("Servo Angle")) -> ()
          }
          frame "Cam Acq" {
            n110 = call "Low-Level Grab.vi"("States"=State_control."Continuous Acquisition ") -> ("error out"=w622:errorcluster, "Image Out"=w623:T29)  [unwired: 8 in, 1 out]
            n111 = call "All object detection ver2.vi"("Image In"=w623, "error in"=w622) -> ("Object detection count"=→"Object detection count":T6, "error out"=w621:errorcluster)  [unwired: 1 out]
          }
          frame "Cam Exit" {
            n112 = call "Low-Level Grab.vi"("States"=State_control."Stop camera") -> ("error out"=w630:errorcluster, "Session Out"=w632:T16)  [unwired: 8 in, 1 out]
            n113 = local write "Servo Angle"(u8 90 ("Servo Angle")) -> ()
            n114 = call "Low-Level Grab.vi"("error in (no error)"=w630, "States"=State_control."Dispose all", "Session In"=w632) -> ("error out"=w629:errorcluster)  [unwired: 6 in, 2 out]
          }
          frame "NavX Calibrate" {
            # "Adds a 15 second delay to the startup process \nfor the NavX to calibrate"
            n115 = Wait (ms)(milliseconds to wait=u32 5000) -> ()  [unwired: 1 out]
          }
        }
        "State logic" <- w167
        "Camera error" <- w151
        n116 = call <vilib>:"Raw Values.vi"("NavX Info In"=w137) -> ("NavX Info Out"=w128:T28)  [unwired: 8 in, 1 out]
        n117 = local read "Manual Zero Yaw"() -> (w131:bool)
        n118 = call <vilib>:"Status.vi"("NavX Info In"=w128) -> ("Status"=→"Status":T3, "NavX Info Out"=w127:T28)  [unwired: 9 in]
        n119 = Or(x=w130, y=w131) -> (x .or. y?=w132:bool)
        n120 = call <vilib>:"YRPHfH.vi"("NavX Info In"=w127) -> ("YRPHfH"=w140:T30, "NavX Info Out"=w139:T28)  [unwired: 3 in]
        n121 = case shown="False" w132 {
          tunnel: [w168 w170] -> w136
          tunnel: w139 -> [w168 w169]
          frame False {
          }
          frame True {
            n122 = call <vilib>:"Zero Yaw.vi"("NavX Info In"=w169) -> ("NavX Info Out"=w170:T28)  [unwired: 10 in]
          }
        }
        n123 = Unbundle By Name(w140) -> ("Yaw"=w134:dbl)
        "Yaw" <- w134
        n124 = call <vilib>:"Displacement.vi"("NavX Info In"=w136) -> ("Displacement"=→"Displacement":T4, "NavX Info Out"=w133:T28)  [unwired: 9 in]
        n125 = call "New motor Control integrated remodeled state based.vi"("Yaw"=w134, "States"=w146) -> ("Speed and distance cluster"=w145:T5)  [unwired: 1 in, 1 out]
        "Speed and distance cluster" <- w145
        n126 = case shown="True" w159 {
          tunnel: w167 -> [w174 w186]
          tunnel: w150 -> [w175 w185]
          tunnel: w156 -> [w173 w181]
          tunnel: [w175 w185] -> w163
          tunnel: [w173 w196] -> w162
          tunnel: [w174 w195] -> w161
          tunnel: w157 -> [_ w194]
          tunnel: w160 -> [_ w193]
          tunnel: w153 -> [w172 w188]
          tunnel: [w172 w188] -> w152
          tunnel: [enum16{"OFF", "ON", "BLINK"}."BLINK" ("GREEN LED State") w182] -> w147
          tunnel: w145 -> [_ w179]
          tunnel: [_ w177] -> w144
          tunnel: w134 -> [_ w176]
          frame False {
          }
          frame True {
            # ">>State Logic Queue Reference >>"
            n127 = Get Queue Status(queue=w185) -> (error out=w184:errorcluster)  [unwired: 2 in, 7 out]
            n128 = local read "DIO 1"() -> (w183:bool)
            n129 = Unbundle(w179) -> (w178:T31)  [unwired: 1 out]
            n130 = case shown="No Error" w184 {
              tunnel: [w197 TLB_MHL_States."Reset" ("Enum")] -> w187
              tunnel: w186 -> [w197 _]
              frame No Error {
              }
              frame Error {
              }
            }
            n131 = Unbundle By Name(w188) -> ("Front Ultrasonic Obstruct"=w189:bool, "Right Ultrasonic Obstruct"=w180:bool)  [unwired: 1 out]
            n132 = Unbundle By Name(w178) -> ("xDistance"=w190:dbl, "yDistance"=w192:dbl, "wDistance"=w191:dbl)
            n133 = case shown="\"Task 3\"" w187 {
              tunnel: w185 -> [w202 w267 w278 w295 w314 w330 w345 w361 w377 w393 _ w417 w439 w452 _ _ _ _]
              tunnel: w181 -> [_ w270 w284 w299 w323 w334 w350 w367 w382 w399 w410 w420 w440 w456 w465 w469 w475 w489]
              tunnel: [w199 w269 w283 w300 w322 w335 w349 w366 w381 w398 w409 w421 w441 w455 w465 w468 w475 w490] -> w196
              tunnel: [w205 TLB_MHL_States."Idle" ("Enum") w286 w301 w319 w338 w352 w365 w383 w397 TLB_MHL_States."Shutdown" ("Enum") w423 w432 w454 TLB_MHL_States."Reset" ("Enum") TLB_MHL_States."Shutdown" ("Enum") TLB_MHL_States."Reset" ("Enum") w486] -> w195
              tunnel: w194 -> [w203 _ _ _ _ _ _ _ _ _ _ _ _ _ _ _ _ _]
              tunnel: w193 -> [w204 _ _ _ _ _ _ _ _ _ _ _ _ _ _ _ _ _]
              tunnel: w183 -> [_ _ w281 w298 w317 _ _ _ _ w396 _ w418 w435 w453 _ _ _ w478]
              tunnel: w192 -> [_ _ w276 _ _ _ w344 w360 _ _ _ _ _ _ _ _ _ _]
              tunnel: w191 -> [_ _ _ _ w312 _ _ _ _ _ _ _ _ _ _ _ _ _]
              tunnel: w190 -> [_ _ _ _ _ _ _ _ w376 _ _ _ _ _ _ _ _ _]
              tunnel: w189 -> [_ _ _ w296 _ w332 _ _ _ w395 _ _ w434 _ _ _ _ _]
              tunnel: [enum16{"OFF", "ON", "BLINK"}."ON" ("GREEN LED State") enum16{"OFF", "ON", "BLINK"}."OFF" ("GREEN LED State") enum16{"OFF", "ON", "BLINK"}."BLINK" ("GREEN LED State") enum16{"OFF", "ON", "BLINK"}."BLINK" ("GREEN LED State") enum16{"OFF", "ON", "BLINK"}."BLINK" ("GREEN LED State") enum16{"OFF", "ON", "BLINK"}."BLINK" ("GREEN LED State") enum16{"OFF", "ON", "BLINK"}."BLINK" ("GREEN LED State") enum16{"OFF", "ON", "BLINK"}."BLINK" ("GREEN LED State") enum16{"OFF", "ON", "BLINK"}."BLINK" ("GREEN LED State") enum16{"OFF", "ON", "BLINK"}."BLINK" ("GREEN LED State") enum16{"OFF", "ON", "BLINK"}."OFF" ("GREEN LED State") enum16{"OFF", "ON", "BLINK"}."BLINK" ("GREEN LED State") enum16{"OFF", "ON", "BLINK"}."BLINK" ("GREEN LED State") enum16{"OFF", "ON", "BLINK"}."BLINK" ("GREEN LED State") _ enum16{"OFF", "ON", "BLINK"}."OFF" ("GREEN LED State") _ _] -> w182
              tunnel: w181 -> [w200 _ _ _ _ _ _ _ _ _ _ _ _ _ _ _ _ _]
              tunnel: w180 -> [_ _ _ _ _ _ _ _ _ _ _ _ _ _ _ _ _ _]
              tunnel: [_ _ _ _ _ _ _ _ _ _ _ _ w430 _ _ _ _ _] -> w177
              tunnel: w176 -> [_ _ _ _ _ _ _ _ _ _ _ _ _ _ _ _ _ w477]
              frame "Idle", Default {
                # ">>State Logic >>"
                n134 = Dequeue Element(queue=w202, timeout in ms (-1)=w204, error in (no error)=w203) -> (element=w206:T7)  [unwired: 3 out]
                "element" <- w206
                n135 = case shown="\"Start Drive Straight\"" w206 {
                  tunnel: [TLB_MHL_States."Idle" ("Enum") TLB_MHL_States."Idle" ("Enum") TLB_MHL_States."Task 1" ("Enum") TLB_MHL_States."Task 2" ("Enum") TLB_MHL_States."Task 3" ("Enum") TLB_MHL_States."Task 4" ("Enum") TLB_MHL_States."Shutdown" ("Enum") TLB_MHL_States."Wall follow mode" ("Enum") TLB_MHL_States."Acquire image" ("Enum") TLB_MHL_States."Autodrive" ("Enum")] -> w205
                  tunnel: w200 -> [w207 w209 w213 w220 w226 w234 w241 w248 w255 w262]
                  tunnel: [w207 w209 w212 w219 w227 w233 w240 w247 w254 w260] -> w199
                  frame "Start Sequence" {
                    # "This event should never be triggered"
                  }
                  frame "Idle", Default {
                    # ">>Action states Queue Reference >>"
                  }
                  frame "Start Task 1" {
                    # ">>Action states Queue Reference >>"
                    # "Action items"
                    n136 = for {
                      shift-right: [w217] -> w212
                      shift-left: w213 -> [w216]
                      tunnel: string[] ["Hardware reset", "Software reset", "Forward", ""] -> [w215] mode=indexing
                      n137 = Enqueue Element(queue=w216, element=w215) -> (queue out=w217:refnum<queue>)  [unwired: 2 in, 2 out]
                    }
                  }
                  frame "Start Task 2" {
                    # ">>Action states Queue Reference >>"
                    # "Action items"
                    n138 = for {
                      shift-right: [w224] -> w219
                      shift-left: w220 -> [w223]
                      tunnel: string[] ["Hardware reset", "Software reset", ""] -> [w222] mode=indexing
                      n139 = Enqueue Element(queue=w223, element=w222) -> (queue out=w224:refnum<queue>)  [unwired: 2 in, 2 out]
                    }
                  }
                  frame "Start Task 3" {
                    # ">>Action states Queue Reference >>"
                    n140 = for {
                      shift-right: [w231] -> w227
                      shift-left: w226 -> [w230]
                      tunnel: string[] ["Hardware reset", "Software reset", ""] -> [w229] mode=indexing
                      n141 = Enqueue Element(queue=w230, element=w229) -> (queue out=w231:refnum<queue>)  [unwired: 2 in, 2 out]
                    }
                  }
                  frame "Start Task 4" {
                    # ">>Action states Queue Reference >>"
                    # "Action items"
                    n142 = for {
                      shift-right: [w238] -> w233
                      shift-left: w234 -> [w237]
                      tunnel: string[] ["Hardware reset", "Software reset", ""] -> [w236] mode=indexing
                      n143 = Enqueue Element(queue=w237, element=w236) -> (queue out=w238:refnum<queue>)  [unwired: 2 in, 2 out]
                    }
                  }
                  frame "Exit" {
                    # ">>Action states Queue Reference >>"
                    # "Action items"
                    n144 = for {
                      shift-right: [w245] -> w240
                      shift-left: w241 -> [w244]
                      tunnel: string[] ["Hardware reset", "Software reset", "Motor Control", "Pre-Exit", "Exit"] -> [w243] mode=indexing
                      n145 = Enqueue Element(queue=w244, element=w243) -> (queue out=w245:refnum<queue>)  [unwired: 2 in, 2 out]
                    }
                  }
                  frame "Wall follow mode" {
                    # ">>Action states Queue Reference >>"
                    # "Action items"
                    n146 = for {
                      shift-right: [w252] -> w247
                      shift-left: w248 -> [w251]
                      tunnel: string[] ["Hardware reset", "Software reset", ""] -> [w250] mode=indexing
                      n147 = Enqueue Element(queue=w251, element=w250) -> (queue out=w252:refnum<queue>)  [unwired: 2 in, 2 out]
                    }
                  }
                  frame "Camera vision" {
                    # ">>Action states Queue Reference >>"
                    # "Action items"
                    n148 = for {
                      shift-right: [w259] -> w254
                      shift-left: w255 -> [w258]
                      tunnel: string[] ["Hardware reset", "Software reset", "Cam Init", "Cam Acq"] -> [w257] mode=indexing
                      n149 = Enqueue Element(queue=w258, element=w257) -> (queue out=w259:refnum<queue>)  [unwired: 2 in, 2 out]
                    }
                  }
                  frame "Start Drive Straight" {
                    # ">>Action states Queue Reference >>"
                    # "Action items"
                    n150 = for {
                      shift-right: [w266] -> w260
                      shift-left: w262 -> [w265]
                      tunnel: string[] ["Hardware reset", "Software reset", "Forward", ""] -> [w264] mode=indexing
                      n151 = Enqueue Element(queue=w265, element=w264) -> (queue out=w266:refnum<queue>)  [unwired: 2 in, 2 out]
                    }
                  }
                }
              }
              frame "Startup" {
                # ">>State Logic >>"
                n152 = Flush Queue(queue=w267) -> ()  [unwired: 1 in, 3 out]
                n153 = for {
                  shift-right: [w274] -> w269
                  shift-left: w270 -> [w275]
                  tunnel: string[] ["Init", "NavX Calibrate", "Software reset", "Hardware reset", "Motor Control"] -> [w273] mode=indexing
                  n154 = Enqueue Element(queue=w275, element=w273) -> (queue out=w274:refnum<queue>)  [unwired: 2 in, 2 out]
                }
              }
              frame "Task 1" {
                # ">>State Logic >>"
                n155 = Greater Or Equal?(x=w276, y=1.2) -> (x >= y?=w279:bool)
                n156 = Or(x=w281, y=w279) -> (x .or. y?=w282:bool)
                n157 = case shown="False" w282 {
                  tunnel: [string[] ["Forward", "Motor Control", "Ultrasonic read"] string[] ["Software reset", "Hardware reset", "Motor Control"]] -> w285
                  frame False {
                  }
                  frame True {
                  }
                }
                n158 = Flush Queue(queue=w278) -> ()  [unwired: 1 in, 3 out]
                n159 = Select(t=TLB_MHL_States."Idle" ("Enum"), s=w282, f=TLB_MHL_States."Task 1" ("Enum")) -> (s? t:f=w286:T8)
                n160 = for {
                  shift-right: [w292] -> w283
                  shift-left: w284 -> [w293]
                  tunnel: w285 -> [w291] mode=indexing
                  n161 = Enqueue Element(queue=w293, element=w291) -> (queue out=w292:refnum<queue>)  [unwired: 2 in, 2 out]
                }
              }
              frame "Task 2" {
                # ">>State Logic >>"
                n162 = Flush Queue(queue=w295) -> ()  [unwired: 1 in, 3 out]
                n163 = case shown="True" w298 {
                  tunnel: [w305 string[] ["Hardware reset", "Software reset", "Motor control"]] -> w297
                  tunnel: w296 -> [w304 _]
                  frame False {
                    n164 = case shown="False" w304 {
                      tunnel: [string[] ["Stop", "Ultrasonic read", "Motor Control"] string[] ["Reverse", "Ultrasonic read", "Motor control"]] -> w305
                      frame False {
                      }
                      frame True {
                      }
                    }
                  }
                  frame True {
                  }
                }
                n165 = Select(t=TLB_MHL_States."Idle" ("Enum"), s=w298, f=TLB_MHL_States."Task 2" ("Enum")) -> (s? t:f=w301:T8)
                n166 = for {
                  shift-right: [w310] -> w300
                  shift-left: w299 -> [w311]
                  tunnel: w297 -> [w309] mode=indexing
                  n167 = Enqueue Element(queue=w311, element=w309) -> (queue out=w310:refnum<queue>)  [unwired: 2 in, 2 out]
                }
              }
              frame "Task 3" {
                n168 = Less Or Equal?(x=w312, y=-1.15) -> (x <= y?=w316:bool)
                n169 = Flush Queue(queue=w314) -> ()  [unwired: 1 in, 3 out]
                n170 = Or(x=w316, y=w317) -> (x .or. y?=w318:bool)
                n171 = case shown="False" w318 {
                  tunnel: [string[] ["Rotate CW", "Motor Control"] string[] ["Software reset", "Hardware reset", "Motor Control"]] -> w324
                  frame False {
                  }
                  frame True {
                  }
                }
                n172 = for {
                  shift-right: [w326] -> w322
                  shift-left: w323 -> [w327]
                  tunnel: w324 -> [w325] mode=indexing
                  n173 = Enqueue Element(queue=w327, element=w325) -> (queue out=w326:refnum<queue>)  [unwired: 2 in, 2 out]
                }
                n174 = Select(t=TLB_MHL_States."Idle" ("Enum"), s=w318, f=TLB_MHL_States."Task 3" ("Enum")) -> (s? t:f=w319:T8)
              }
              frame "Task 4" {
                n175 = Flush Queue(queue=w330) -> ()  [unwired: 1 in, 3 out]
                n176 = case shown="True" w332 {
                  tunnel: [string[] ["Forward", "Ultrasonic read", "Motor Control"] string[] ["Stop", "Hardware reset", "Software reset", "Motor Control"]] -> w333
                  frame False {
                  }
                  frame True {
                  }
                }
                n177 = for {
                  shift-right: [w342] -> w335
                  shift-left: w334 -> [w343]
                  tunnel: w333 -> [w341] mode=indexing
                  n178 = Enqueue Element(queue=w343, element=w341) -> (queue out=w342:refnum<queue>)  [unwired: 2 in, 2 out]
                }
                n179 = Select(t=TLB_MHL_States."Task 4a" ("Enum"), s=w332, f=TLB_MHL_States."Task 4" ("Enum")) -> (s? t:f=w338:T8)
              }
              frame "Task 4a" {
                n180 = Greater Or Equal?(x=w344, y=0.5) -> (x >= y?=w348:bool)
                n181 = Flush Queue(queue=w345) -> ()  [unwired: 1 in, 3 out]
                n182 = case shown="True" w348 {
                  tunnel: [string[] ["Right", "Motor Control"] string[] ["Stop", "Hardware reset", "Software reset", "Motor Control"]] -> w351
                  frame False {
                  }
                  frame True {
                  }
                }
                n183 = for {
                  shift-right: [w358] -> w349
                  shift-left: w350 -> [w359]
                  tunnel: w351 -> [w357] mode=indexing
                  n184 = Enqueue Element(queue=w359, element=w357) -> (queue out=w358:refnum<queue>)  [unwired: 2 in, 2 out]
                }
                n185 = Select(t=TLB_MHL_States."Task 4b" ("Enum"), s=w348, f=TLB_MHL_States."Task 4a" ("Enum")) -> (s? t:f=w352:T8)
              }
              frame "Task 4b" {
                n186 = Flush Queue(queue=w361) -> ()  [unwired: 1 in, 3 out]
                n187 = Greater Or Equal?(x=w360, y=0.75) -> (x >= y?=w363:bool)
                n188 = case shown="False" w363 {
                  tunnel: [string[] ["Forward", "Motor control"] string[] ["Stop", "Hardware reset", "Software reset"]] -> w368
                  frame False {
                  }
                  frame True {
                  }
                }
                n189 = for {
                  shift-right: [w374] -> w366
                  shift-left: w367 -> [w375]
                  tunnel: w368 -> [w373] mode=indexing
                  n190 = Enqueue Element(queue=w375, element=w373) -> (queue out=w374:refnum<queue>)  [unwired: 2 in, 2 out]
                }
                n191 = Select(t=TLB_MHL_States."Task 4c" ("Enum"), s=w363, f=TLB_MHL_States."Task 4b" ("Enum")) -> (s? t:f=w365:T8)
              }
              frame "Task 4c" {
                n192 = Flush Queue(queue=w377) -> ()  [unwired: 1 in, 3 out]
                n193 = Less Or Equal?(x=w376, y=-0.65) -> (x <= y?=w379:bool)
                n194 = case shown="False" w379 {
                  tunnel: [string[] ["Left", "Motor Control"] string[] ["Stop", "Hardware reset", "Software reset", "Motor Control"]] -> w384
                  frame False {
                  }
                  frame True {
                  }
                }
                n195 = for {
                  shift-right: [w390] -> w381
                  shift-left: w382 -> [w391]
                  tunnel: w384 -> [w389] mode=indexing
                  n196 = Enqueue Element(queue=w391, element=w389) -> (queue out=w390:refnum<queue>)  [unwired: 2 in, 2 out]
                }
                n197 = Select(t=TLB_MHL_States."Task 4d" ("Enum"), s=w379, f=TLB_MHL_States."Task 4c" ("Enum")) -> (s? t:f=w383:T8)
              }
              frame "Task 4d" {
                n198 = Flush Queue(queue=w393) -> ()  [unwired: 1 in, 3 out]
                n199 = Or(x=w396, y=w395) -> (x .or. y?=w394:bool)
                n200 = case shown="True" w394 {
                  tunnel: [string[] ["Forward", "Ultrasonic Read", "Motor Control"] string[] ["Stop", "Hardware reset", "Software reset", "Motor Control"]] -> w400
                  frame False {
                  }
                  frame True {
                  }
                }
                n201 = for {
                  shift-right: [w406] -> w398
                  shift-left: w399 -> [w407]
                  tunnel: w400 -> [w405] mode=indexing
                  n202 = Enqueue Element(queue=w407, element=w405) -> (queue out=w406:refnum<queue>)  [unwired: 2 in, 2 out]
                }
                n203 = Select(t=TLB_MHL_States."Idle" ("Enum"), s=w394, f=TLB_MHL_States."Task 4d" ("Enum")) -> (s? t:f=w397:T8)
              }
              frame "Reset" {
                n204 = for {
                  shift-right: [w414] -> w409
                  shift-left: w410 -> [w415]
                  tunnel: string[] ["Software reset", "Hardware reset", "Motor Control"] -> [w413] mode=indexing
                  n205 = Enqueue Element(queue=w415, element=w413) -> (queue out=w414:refnum<queue>)  [unwired: 2 in, 2 out]
                }
              }
              frame "Wall follow mode" {
                n206 = Flush Queue(queue=w417) -> ()  [unwired: 1 in, 3 out]
                n207 = case shown="False" w418 {
                  tunnel: [string[] ["IR Sensor Read", "Calculate", "Forward", "Motor Control"] string[] ["Hardware reset", "Software reset", "Motor Control"]] -> w419
                  frame False {
                  }
                  frame True {
                  }
                }
                n208 = for {
                  shift-right: [w428] -> w421
                  shift-left: w420 -> [w429]
                  tunnel: w419 -> [w427] mode=indexing
                  n209 = Enqueue Element(queue=w429, element=w427) -> (queue out=w428:refnum<queue>)  [unwired: 2 in, 2 out]
                }
                n210 = Select(t=TLB_MHL_States."Idle" ("Enum"), s=w418, f=TLB_MHL_States."Wall follow mode" ("Enum")) -> (s? t:f=w423:T8)
              }
              frame "Autodrive" {
                # ">>>Return to idle event>>>"
                n211 = Flush Queue(queue=w439) -> ()  [unwired: 1 in, 3 out]
                n212 = Boolean To (0,1)(Boolean=w435) -> (0, 1=w437:i16)
                n213 = Boolean To (0,1)(Boolean=w434) -> (0, 1=w436:i16)
                n214 = formula code="int8  out;\nif (detect == 0 && stop == 0)\nout = 0;\n\nelse if (detect == 1 && stop == 0)\nout = 1;\n\nelse if (detect == 0 && stop == 1)\nout = 2;\n\nelse\nout = 0;"("stop"=w437, "detect"=w436) -> ("out"=w430:i8)
                n215 = case shown="0, Default" w430 {
                  tunnel: [string[] ["Forward", "Ultrasonic read"] string[] ["Hardware reset", "Software reset", "Rotate Clockwise", ""] string[] ["Stop", "Hardware reset", "Software reset", "Motor Control"]] -> w433
                  frame 0, Default {
                  }
                  frame 1 {
                  }
                  frame 2 {
                  }
                }
                n216 = call "Servo State FGV.vi"("Init/Read/Write State"=States_for_Action_Engine."Write", "Servo State"=w430) -> ()  [unwired: 1 in, 2 out]
                n217 = for {
                  shift-right: [w449] -> w441
                  shift-left: w440 -> [w450]
                  tunnel: w433 -> [w448] mode=indexing
                  n218 = Enqueue Element(queue=w450, element=w448) -> (queue out=w449:refnum<queue>)  [unwired: 2 in, 2 out]
                }
                n219 = case shown="2" w430 {
                  tunnel: [TLB_MHL_States."Autodrive" ("Enum") TLB_MHL_States."Autodrive a" ("Enum") TLB_MHL_States."Idle" ("Enum")] -> w432
                  frame 0, Default {
                  }
                  frame 1 {
                  }
                  frame 2 {
                  }
                }
              }
              frame "Acquire image" {
                n220 = Flush Queue(queue=w452) -> ()  [unwired: 1 in, 3 out]
                n221 = case shown="True" w453 {
                  tunnel: [string[] ["Cam Acq"] string[] ["Hardware reset", "Software reset", "Cam Exit", ""]] -> w457
                  frame False {
                  }
                  frame True {
                  }
                }
                n222 = for {
                  shift-right: [w463] -> w455
                  shift-left: w456 -> [w464]
                  tunnel: w457 -> [w462] mode=indexing
                  n223 = Enqueue Element(queue=w464, element=w462) -> (queue out=w463:refnum<queue>)  [unwired: 2 in, 2 out]
                }
                n224 = Select(t=TLB_MHL_States."Idle" ("Enum"), s=w453, f=TLB_MHL_States."Acquire image" ("Enum")) -> (s? t:f=w454:T8)
              }
              frame "Processing" {
              }
              frame "Shutdown" {
                # ">>State Logic >>"
                n225 = for {
                  shift-right: [w473] -> w468
                  shift-left: w469 -> [w474]
                  tunnel: string[] ["Software reset", "Hardware reset", "Motor Control", "Cam Exit", "Pre-Exit", "Exit"] -> [w472] mode=indexing
                  n226 = Enqueue Element(queue=w474, element=w472) -> (queue out=w473:refnum<queue>)  [unwired: 2 in, 2 out]
                }
              }
              frame "None" {
              }
              frame "Autodrive a" {
                n227 = Greater Or Equal?(x=w477, y=80.0) -> (x >= y?=w479:bool)
                n228 = Or(x=w478, y=w479) -> (x .or. y?=w480:bool)
                n229 = case shown="True" w480 {
                  tunnel: [string[] ["Rotate CW", "Ultrasonic read", ""] string[] ["Stop", "Hardware reset", "Software reset", ""]] -> w488
                  frame False {
                  }
                  frame True {
                  }
                }
                n230 = for {
                  shift-right: [w494] -> w490
                  shift-left: w489 -> [w495]
                  tunnel: w488 -> [w493] mode=indexing
                  n231 = Enqueue Element(queue=w495, element=w493) -> (queue out=w494:refnum<queue>)  [unwired: 2 in, 2 out]
                }
                n232 = Or(x=w478, y=w479) -> (x .or. y?=w481:bool)
                n233 = Select(t=TLB_MHL_States."Idle" ("Enum"), s=w478, f=TLB_MHL_States."Autodrive" ("Enum")) -> (s? t:f=w484:T8)
                n234 = Select(t=w484, s=w481, f=TLB_MHL_States."Autodrive a" ("Enum")) -> (s? t:f=w486:T8)
              }
            }
          }
        }
        n235 = call "Servo State FGV.vi"("Init/Read/Write State"=States_for_Action_Engine."Read") -> ("Output"=→"Output":dbl)  [unwired: 2 in, 1 out]
        n236 = local write "GREEN LED State"(w147) -> ()
        "Decision" <- w143
      }
      n237 = call <vilib>:"DIO Close.vi"("DIO Info In"=w11) -> ()  [unwired: 10 in, 1 out]
      n238 = call <vilib>:"DIO Close.vi"("error in (no error)"=w28, "DIO Info In"=w34) -> ()  [unwired: 9 in, 1 out]
      n239 = call <vilib>:"DIO Close.vi"("error in (no error)"=w26, "DIO Info In"=w30) -> ()  [unwired: 9 in, 1 out]
      n240 = call <vilib>:"DIO Close.vi"("error in (no error)"=w16, "DIO Info In"=w21) -> ()  [unwired: 9 in, 1 out]
      n241 = call <vilib>:"DIO Close.vi"("error in (no error)"=w14, "DIO Info In"=w20) -> ()  [unwired: 9 in, 1 out]
      n242 = while {
        shift-right: [w109] -> _
        shift-left: _ -> [w110]
        shift-right: [w108] -> _
        shift-left: _ -> [w107]
        stop <- w116 stop-if-true
        (unwired) TRUE
        # "LED Blinker Loop"
        n243 = case shown="\"BLINK\"" "GREEN LED State" {
          tunnel: [FALSE TRUE w124] -> w112
          tunnel: w110 -> [_ _ w124]
          tunnel: [_ _ w125] -> w109
          frame "OFF", Default {
          }
          frame "ON" {
          }
          frame "BLINK" {
            n244 = Not(x=w124) -> (.not. x?=w125:bool)
          }
        }
        n245 = case shown="\"OFF\", Default" "RED LED State" {
          tunnel: [FALSE TRUE w120] -> w111
          tunnel: [_ _ w121] -> w108
          tunnel: w107 -> [_ _ w120]
          frame "OFF", Default {
          }
          frame "ON" {
          }
          frame "BLINK" {
            n246 = Not(x=w120) -> (.not. x?=w121:bool)
          }
        }
        n247 = local write "Green LED"(w112) -> ()
        n248 = local write "Red LED"(w111) -> ()
        n249 = call "FGV Bool.vi"("Init/Read/Write State"=States_for_Action_Engine."Read") -> ("Output node"=w116:bool)  [unwired: 2 in, 1 out]
        n250 = Wait (ms)(milliseconds to wait=u32 500) -> ()  [unwired: 1 out]
      }
      n251 = Merge Errors "Merge Errors"(w60, w59) -> (w41:errorcluster)
      n252 = Merge Errors(w45, w41) -> (w36:errorcluster)
      n253 = Destroy User Event(user event=w63, error in=w36) -> ()  [unwired: 1 out]
      n254 = Destroy User Event(user event=w64, error in=w36) -> ()  [unwired: 1 out]
      n255 = Unregister For Events(event registration refnum=w55, error in=w36) -> ()  [unwired: 1 out]
      n256 = Release Queue(queue=w38, error in (no error)=w36) -> (error out=→"error out":errorcluster)  [unwired: 1 in, 2 out]
      n257 = call <vilib>:"NavX Close.vi"("NavX Info In"=w10) -> ()  [unwired: 10 in, 1 out]
      n258 = Release Queue(queue=w54, error in (no error)=w36) -> ()  [unwired: 1 in, 3 out]
    }
    frame #2 {
      (unwired) T18."INIT" ("States")
      n259 = call "New motor Control integrated remodeled state based.vi"() -> ()  [unwired: 3 in, 2 out]
    }
    frame #3 {
    }
  }
